vi "Formatted Delayed Coordinates and Date Time.VI"() -> ()   [LabVIEW 2012]
panel:
  out "String":string="Run To Select A File"
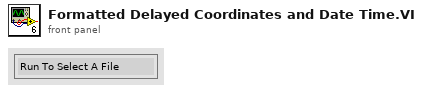
[diagram p1: front panel]
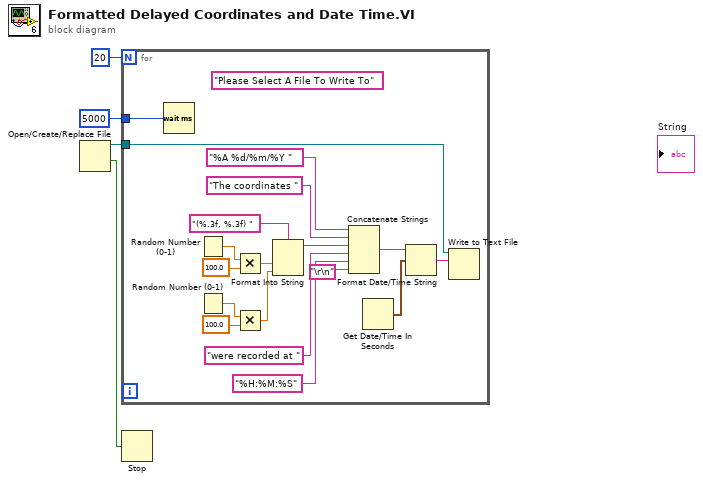
[diagram p0: block diagram]
diagram:
  n1 = Open/Create/Replace File() -> (refnum out=w3:refnum<file>, cancelled=w2:bool)  [unwired: 6 in, 1 out]
  n2 = for {
    N: 20 -> [_]
    tunnel: w3 -> [w15]
    tunnel: u32 5000 ("millisecond multiple") -> [w5]
    (unwired) "Please Select A File To Write To"
    n3 = Wait (ms)(milliseconds to wait=w5) -> ()  [unwired: 1 out]
    n4 = Random Number (0-1)() -> (number: 0 to 1=w22:dbl)
    n5 = Random Number (0-1)() -> (number: 0 to 1=w21:dbl)
    n6 = Multiply(x=w22, y=100.0) -> (x*y=w18:dbl)
    n7 = Multiply(x=w21, y=100.0) -> (x*y=w17:dbl)
    n8 = Format Into String(format string="(%.3f, %.3f) ", w18, w17) -> (resulting string=w12:string)  [unwired: 2 in, 1 out]
    n9 = Concatenate Strings("%A %d/%m/%Y ", "The coordinates ", w12, "were recorded at ", "%H:%M:%S", "\r\n") -> (w8:string)
    n10 = Get Date/Time In Seconds() -> (seconds since 1Jan1904=w14:timestamp)
    n11 = Format Date/Time String(time format string (%c)=w8, seconds (now)=w14) -> (date/time string=w7:string)  [unwired: 1 in]
    n12 = Write to Text File(file (use dialog)=w15, text=w7) -> ()  [unwired: 2 in, 3 out]
  }
  n13 = Stop(stop? (T)=w2) -> ()
